vi "Ejercicios 1 a 3 para el reporte 2.vi"() -> ()   [LabVIEW 2014]
uses:
  <vilib>/Analysis/2dsp.llb/Real FFT.vi
  <vilib>/measure/NI_MABase.lvlib
  <vilib>/Analysis/NI_AALPro.lvlib
panel:
  out "error":i32
  in  "FFT size":i32=-1
  in  "shift?":bool
  out "Waveform Graph 2":dbl[](graph)
  out "Waveform Graph":waveform(dbl)(graph)
  out "error out 2":errorcluster
  in  "stop":bool
  in  "reset signal":bool
  in  "signal type":T1(ring)
  in  "offset":dbl format="%0.2p"
  out "signal out":waveform(dbl)
  out "phase out":dbl format="%.2p"
  in  "square wave duty cycle (%)":dbl=50.0 format="%0.2f"
  in  "sampling info":cluster{"Fs":dbl, "#s":dbl}={"Fs"=1000.0, "#s"=1000.0} {"Fs" format="%.2p"}
  in  "error in (no error)":errorcluster
  in  "phase":dbl format="%.2p"
  in  "amplitude":dbl=1.0 format="%0.2p"
  in  "frequency":dbl=10.0 format="%0.2p"
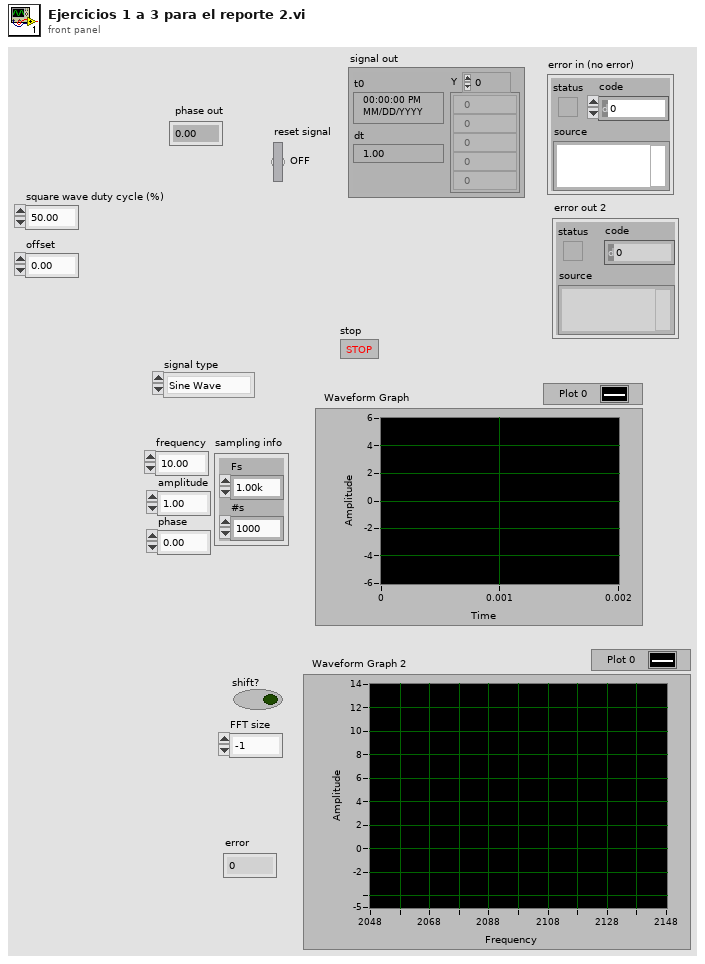
[diagram p1: front panel]
types:
  T1 = enum16{"Sine Wave", "Triangle Wave", "Square Wave", "Sawtooth Wave"}
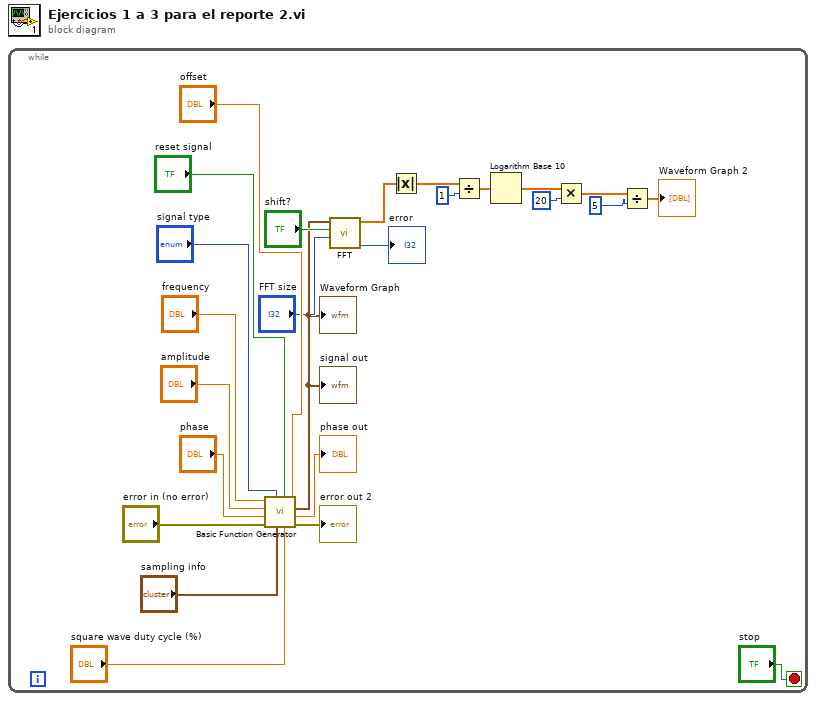
[diagram p0: block diagram]
diagram:
  n1 = while {
    stop <- "stop" stop-if-true
    n2 = call <vilib>:"Basic Function Generator.vi"("offset"="offset", "square wave duty cycle (%)"="square wave duty cycle (%)", "reset signal"="reset signal", "sampling info"="sampling info", "signal type"="signal type", "error in (no error)"="error in (no error)", "phase"="phase", "amplitude"="amplitude", "frequency"="frequency") -> ("error out"=→"error out 2":errorcluster, "phase out"=→"phase out":dbl, "signal out"=w10:waveform(dbl))
    "signal out" <- w10
    "Waveform Graph" <- w10
    n3 = call-poly <vilib>:"FFT.vi"("FFT size"="FFT size", "shift?"="shift?", "X"=w10) -> ("error"=→"error":i32, "FFT {X}"=w5:cdb[])  [unwired: 7 in]
    n4 = Absolute Value(x=w5) -> (abs(x)=w6:dbl[])
    n5 = Divide(x=w6, y=1) -> (x/y=w7:dbl[])
    n6 = Logarithm Base 10(1:w7) -> (0:w8:dbl[])
    n7 = Multiply(x=w8, y=20) -> (x*y=w3:dbl[])
    n8 = Divide(x=w3, y=5) -> (x/y=→"Waveform Graph 2":dbl[])
  }
